vi "gmail.vi"(0 "Send?":bool, 1 "Ring":u16(ring) items=["Start", "Stop", "Each"], 3 "Attachment - Optional":path) -> ()   [LabVIEW 2010]
panel:
  in  "CC (Carbon Copy Recipient - Optional)":string
  in  "Port":i32=587
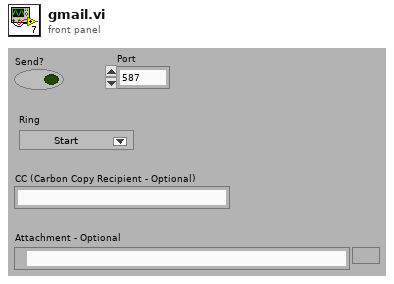
[diagram p1: front panel]
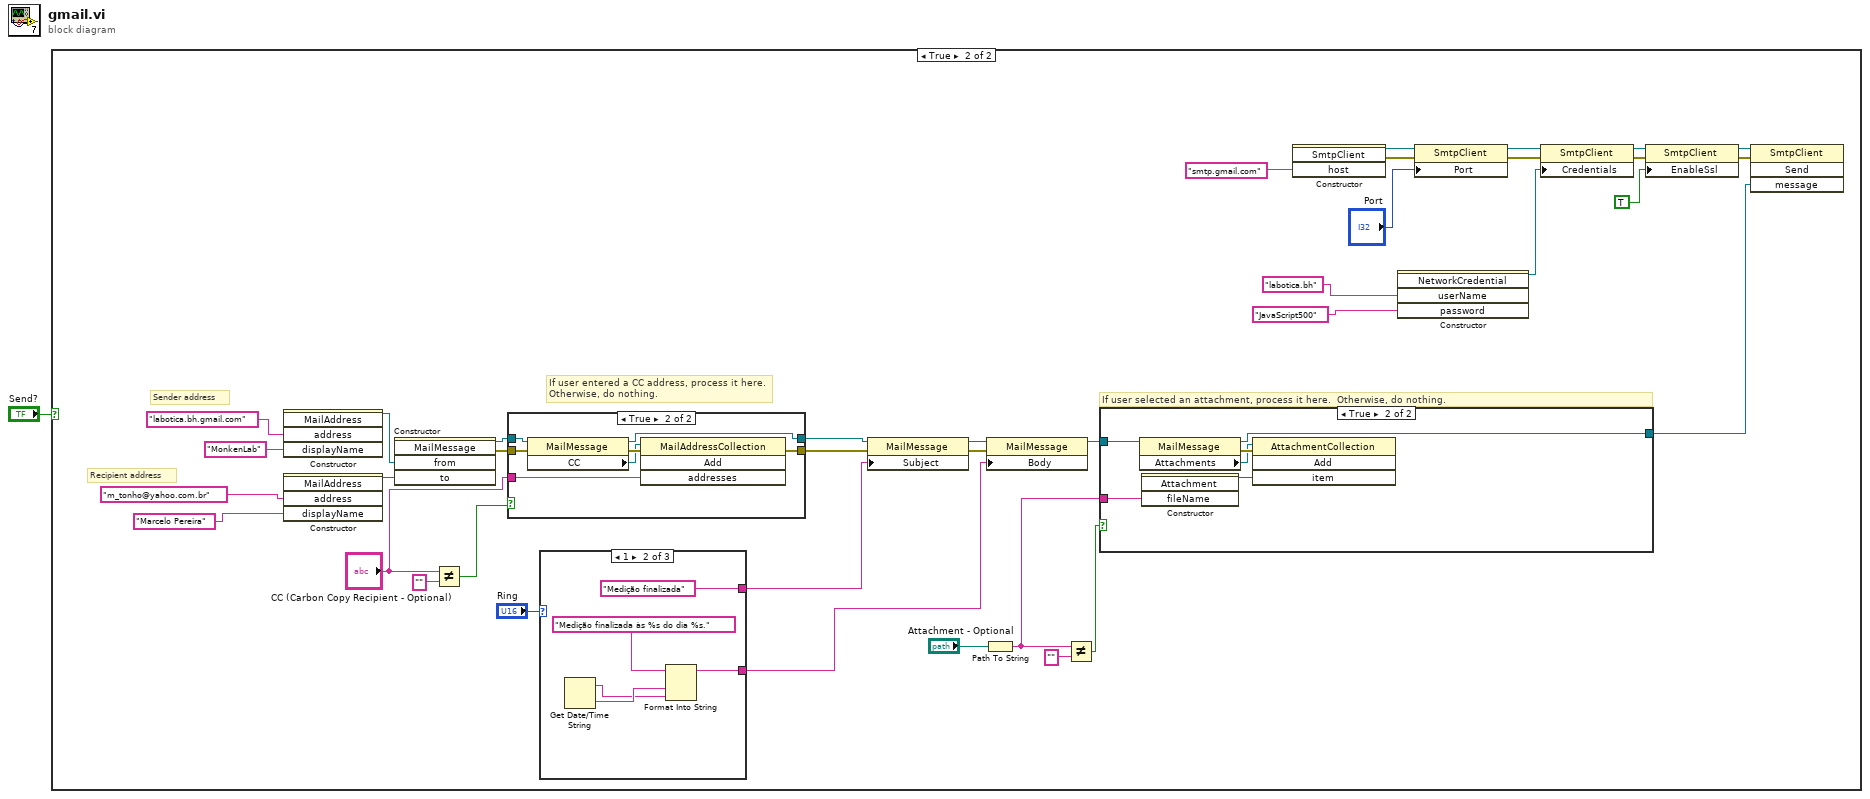
[diagram p0: block diagram]
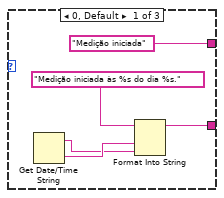
[diagram p3: hidden frame]
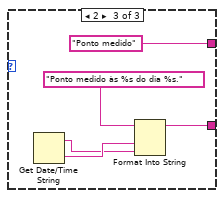
[diagram p4: hidden frame]
diagram:
  n1 = case shown="True" "Send?" {
    frame False {
    }
    frame True {
      # "Recipient address"
      # "Sender address"
      # "If user selected an attachment, process it here.  Otherwise, do nothing."
      # "If user entered a CC address, process it here.\nOtherwise, do nothing."
      n2 = constructor class="MailAddress"("address"="labotica.bh.gmail.com", "displayName"="MonkenLab") -> (reference out=w38:refnum<k24>)  [unwired: 3 in, 4 out]
      n3 = constructor class="MailAddress"("address"="m_tonho@yahoo.com.br", "displayName"="Marcelo Pereira") -> (reference out=w39:refnum<k24>)  [unwired: 3 in, 4 out]
      n4 = constructor class="MailMessage"("from"=w38, "to"=w39) -> (reference out=w16:refnum<k24>, error out=w15:errorcluster)  [unwired: 3 in, 3 out]
      n5 = Not Equal?(x="CC (Carbon Copy Recipient - Optional)", y="") -> (x != y?=w18:bool)
      n6 = case shown="True" w18 {
        tunnel: "CC (Carbon Copy Recipient - Optional)" -> [_ w61]
        tunnel: w16 -> [w56 w60]
        tunnel: w15 -> [w55 w59]
        tunnel: [w56 w58] -> w14
        tunnel: [w55 w57] -> w13
        frame False {
        }
        frame True {
          n7 = property class="MailMessage"(reference=w60, error in=w59) -> (reference out=w58:refnum<k24>, error out=w63:errorcluster, "CC"=w62:refnum<k24>)
          n8 = invoke class="MailAddressCollection" method="Add"(reference=w62, error in=w63, "addresses"=w61) -> (error out=w57:errorcluster)  [unwired: 1 in, 3 out]
        }
      }
      n9 = case shown="1" "Ring" {
        tunnel: ["Medição iniciada" "Medição finalizada" "Ponto medido"] -> w6
        tunnel: [w40 w45 w50] -> w5
        frame 0, Default {
          n10 = Get Date/Time String() -> (date string=w42:string, time string=w43:string)  [unwired: 3 in]
          n11 = Format Into String(format string="Medição iniciada às %s do dia %s.", w43, w42) -> (resulting string=w40:string)  [unwired: 2 in, 1 out]
        }
        frame 1 {
          n12 = Get Date/Time String() -> (date string=w47:string, time string=w48:string)  [unwired: 3 in]
          n13 = Format Into String(format string="Medição finalizada às %s do dia %s.", w48, w47) -> (resulting string=w45:string)  [unwired: 2 in, 1 out]
        }
        frame 2 {
          n14 = Get Date/Time String() -> (date string=w52:string, time string=w53:string)  [unwired: 3 in]
          n15 = Format Into String(format string="Ponto medido às %s do dia %s.", w53, w52) -> (resulting string=w50:string)  [unwired: 2 in, 1 out]
        }
      }
      n16 = property class="MailMessage"(reference=w14, error in=w13, "Subject"=w6) -> (reference out=w36:refnum<k24>, error out=w37:errorcluster)
      n17 = Path To String(path="Attachment - Optional") -> (string=w20:string)
      n18 = property class="MailMessage"(reference=w36, error in=w37, "Body"=w5) -> (reference out=w25:refnum<k24>)  [unwired: 1 out]
      n19 = Not Equal?(x=w20, y="") -> (x != y?=w21:bool)
      n20 = case shown="True" w21 {
        tunnel: w25 -> [w64 w67]
        tunnel: [w64 w66] -> w24
        tunnel: w20 -> [_ w65]
        frame False {
        }
        frame True {
          n21 = property class="MailMessage"(reference=w67) -> (reference out=w66:refnum<k24>, error out=w70:errorcluster, "Attachments"=w68:refnum<k24>)  [unwired: 1 in]
          n22 = constructor class="Attachment"("fileName"=w65) -> (reference out=w69:refnum<k24>)  [unwired: 3 in, 3 out]
          n23 = invoke class="AttachmentCollection" method="Add"(reference=w68, error in=w70, "item"=w69) -> ()  [unwired: 1 in, 4 out]
        }
      }
      n24 = constructor class="SmtpClient"("host"="smtp.gmail.com") -> (reference out=w33:refnum<k24>, error out=w29:errorcluster)  [unwired: 3 in, 2 out]
      n25 = constructor class="NetworkCredential"("userName"="labotica.bh", "password"="JavaScript500") -> (reference out=w34:refnum<k24>)  [unwired: 3 in, 4 out]
      n26 = property class="SmtpClient"(reference=w33, error in=w29, "Port"="Port") -> (reference out=w32:refnum<k24>, error out=w28:errorcluster)
      n27 = property class="SmtpClient"(reference=w32, error in=w28, "Credentials"=w34) -> (reference out=w31:refnum<k24>, error out=w27:errorcluster)
      n28 = property class="SmtpClient"(reference=w31, error in=w27, "EnableSsl"=TRUE) -> (reference out=w30:refnum<k24>, error out=w26:errorcluster)
      n29 = invoke class="SmtpClient" method="Send"(reference=w30, error in=w26, "message"=w24) -> ()  [unwired: 1 in, 4 out]
    }
  }
